vi "Cycle Start.vi"(8 "error in (no error)":errorcluster, 11 "Automation Controller in":refnum<class "Automation Controller.lvclass">) -> (0 "error out":errorcluster, 3 "Automation Controller out":refnum<class "Automation Controller.lvclass">)   [LabVIEW 2024, in "Automation Controller.lvlib" / "Automation Controller.lvclass"]
uses:
  Automation Controller.lvclass
  Automation Controller.lvclass/Automation Controller.ctl
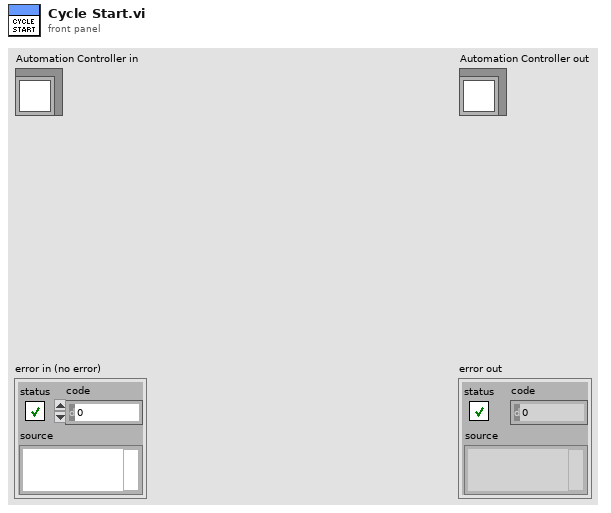
[diagram p1: front panel]
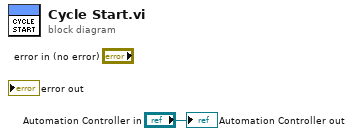
[diagram p0: block diagram]
diagram:
  "Automation Controller out" <- "Automation Controller in"
